vi "Documation.vi"(0 "Max Scale":dbl, 1 "File Nm and format":string, 2 "User/System":string, 3 "Temp":dbl, 4 "Min Scale":dbl) -> (5 "Table":string[][](table))   [LabVIEW 2016]
uses:
  Global Flir-Ax8.vi
  <vilib>/Utility/file.llb/Write Delimited Spreadsheet (string).vi
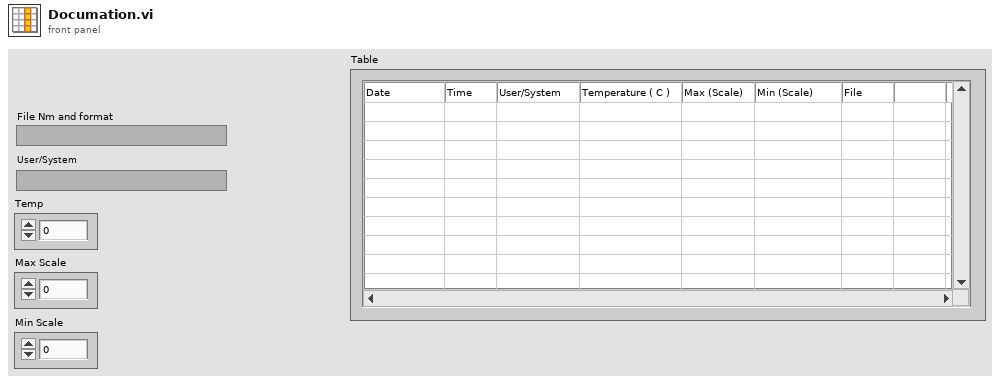
[diagram p1: front panel]
types:
  T1 = enum16{"Check existing file", "create a new file", "write to file", "exit"}
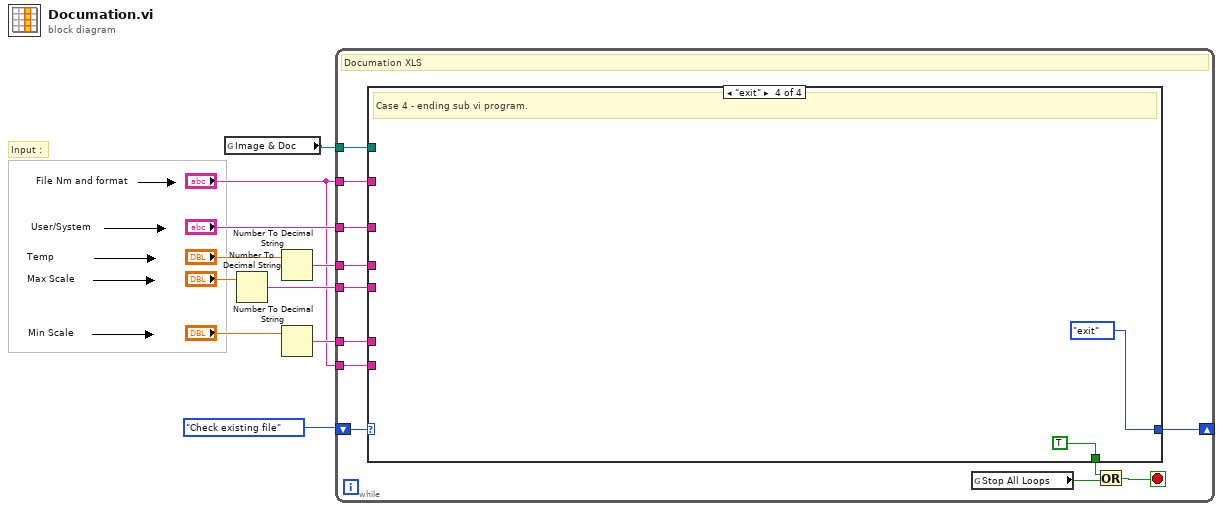
[diagram p0: block diagram]
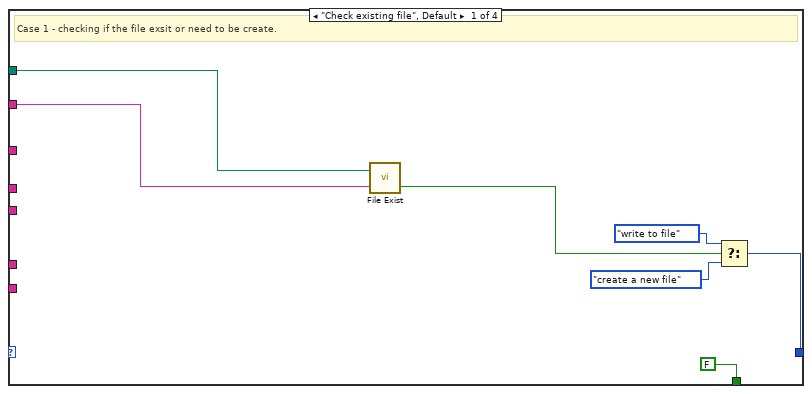
[diagram p2: hidden frame]
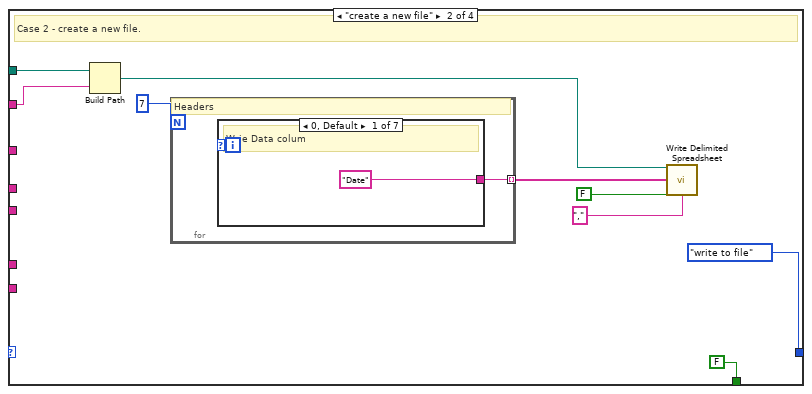
[diagram p3: hidden frame]
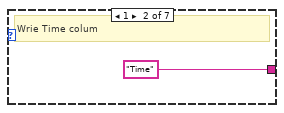
[diagram p4: hidden frame]
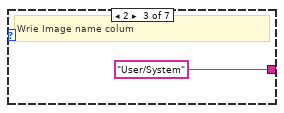
[diagram p5: hidden frame]
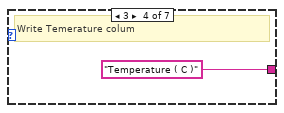
[diagram p6: hidden frame]
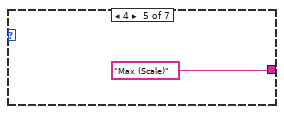
[diagram p7: hidden frame]
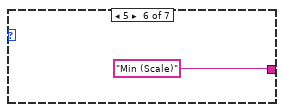
[diagram p8: hidden frame]
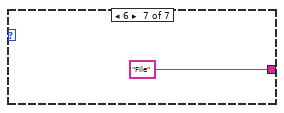
[diagram p9: hidden frame]
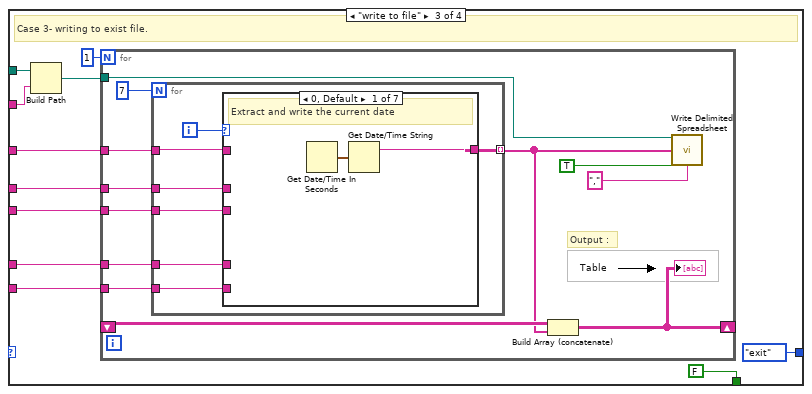
[diagram p10: hidden frame]
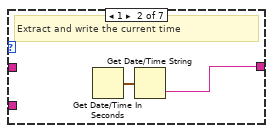
[diagram p11: hidden frame]
diagram:
  # "Input :"
  n1 = global read "Global Flir-Ax8.vi" "Image & Doc"() -> (w1:path)
  n2 = Number To Decimal String(number="Max Scale") -> (decimal integer string=w5:string)  [unwired: 1 in]
  n3 = Number To Decimal String(number="Temp") -> (decimal integer string=w8:string)  [unwired: 1 in]
  n4 = Number To Decimal String(number="Min Scale") -> (decimal integer string=w3:string)  [unwired: 1 in]
  n5 = while {
    shift-right: [w21] -> _
    shift-left: T1."Check existing file" -> [w22]
    tunnel: "User/System" -> [w20]
    tunnel: w1 -> [w19]
    tunnel: "File Nm and format" -> [w18]
    tunnel: w8 -> [w17]
    tunnel: w5 -> [w16]
    tunnel: w3 -> [w15]
    tunnel: "File Nm and format" -> [w14]
    stop <- w11 stop-if-true
    # "Documation XLS"
    n6 = case "Case 1 - checking if the file exsit or need to be create." shown="\"exit\"" w22 {
      tunnel: [w29 T1."write to file" T1."exit" T1."exit"] -> w21
      tunnel: w20 -> [_ _ w57 _]
      tunnel: w19 -> [w28 w34 w56 _]
      tunnel: w18 -> [w24 w33 w55 _]
      tunnel: w17 -> [_ _ w54 _]
      tunnel: w16 -> [_ _ w51 _]
      tunnel: w15 -> [_ _ w50 _]
      tunnel: w14 -> [_ _ w49 _]
      tunnel: [FALSE FALSE FALSE TRUE] -> w12
      frame "Check existing file", Default {
        # "Case 1 - checking if the file exsit or need to be create."
        n7 = call "File Exist.vi"("File Nm"=w24, "File path"=w28) -> ("File Exists"=w25:bool)  [unwired: 1 out]
        n8 = Select(t=T1."write to file", s=w25, f=T1."create a new file") -> (s? t:f=w29:T1)
      }
      frame "create a new file" {
        # "Case 2 - create a new file."
        n9 = Build Path(base path=w34, name or relative path=w33) -> (appended path=w35:path)
        n10 = for {
          N: 7 -> [_]
          tunnel: [w39] -> w38 mode=indexing
          i -> [w40]
          # "Headers"
          n11 = case shown="0, Default" w40 {
            tunnel: ["Date" "Time" "User/System" "Temperature ( C )" "Max (Scale)" "Min (Scale)" "File"] -> w39
            frame 0, Default {
              # "Wrie Data colum"
            }
            frame 1 {
              # "Wrie Time colum"
            }
            frame 2 {
              # "Wrie Image name colum"
            }
            frame 3 {
              # "Write Temerature colum"
            }
            frame 4 {
            }
            frame 5 {
            }
            frame 6 {
            }
          }
        }
        n12 = call-poly <vilib>:"Write Delimited Spreadsheet.vi"("file path (dialog if empty)"=w35, "1D data"=w38, "append to file? (new file:F)"=FALSE, "delimiter (\\t)"="," ("delimiter (\\t)")) -> ()  [unwired: 10 in, 2 out]
      }
      frame "write to file" {
        # "Case 3- writing to exist file."
        n13 = Build Path(base path=w56, name or relative path=w55) -> (appended path=w58:path)
        n14 = for {
          N: 1 -> [_]
          tunnel: w58 -> [w68]
          tunnel: w57 -> [w67]
          tunnel: w54 -> [w66]
          shift-right: [w59] -> _
          shift-left: _ -> [w64]
          tunnel: w51 -> [w62]
          tunnel: w50 -> [w61]
          tunnel: w49 -> [w60]
          # "Output :"
          n15 = for {
            N: 7 -> [_]
            tunnel: [w76] -> w63 mode=indexing
            tunnel: w67 -> [w75]
            tunnel: w66 -> [w74]
            tunnel: w62 -> [w73]
            tunnel: w61 -> [w72]
            tunnel: w60 -> [w71]
            i -> [w77]
            n16 = case shown="0, Default" w77 {
              tunnel: [w78 w80 w82 w83 w84 w85 w86] -> w76
              tunnel: w75 -> [_ _ w82 _ _ _ _]
              tunnel: w74 -> [_ _ _ w83 _ _ _]
              tunnel: w73 -> [_ _ _ _ w84 _ _]
              tunnel: w72 -> [_ _ _ _ _ w85 _]
              tunnel: w71 -> [_ _ _ _ _ _ w86]
              frame 0, Default {
                # "Extract and write the current date"
                n17 = Get Date/Time In Seconds() -> (seconds since 1Jan1904=w79:timestamp)
                n18 = Get Date/Time String(seconds (now)=w79) -> (date string=w78:string)  [unwired: 2 in, 1 out]
              }
              frame 1 {
                # "Extract and write the current time"
                n19 = Get Date/Time In Seconds() -> (seconds since 1Jan1904=w81:timestamp)
                n20 = Get Date/Time String(seconds (now)=w81) -> (time string=w80:string)  [unwired: 2 in, 1 out]
              }
              frame 2 {
                # "insert image name"
              }
              frame 3 {
                # "insert the overstep temerature"
              }
              frame 4 {
                # "insert the max scale temperature"
              }
              frame 5 {
                # "insert the min scale temperature"
              }
              frame 6 {
                # "insert the file name"
              }
            }
          }
          n21 = Build Array (concatenate)(w64, w63) -> (w59:string[][])
          "Table" <- w59
          n22 = call-poly <vilib>:"Write Delimited Spreadsheet.vi"("file path (dialog if empty)"=w68, "1D data"=w63, "append to file? (new file:F)"=TRUE, "delimiter (\\t)"="," ("delimiter (\\t)")) -> ()  [unwired: 10 in, 2 out]
        }
      }
      frame "exit" {
        # "Case 4 - ending sub vi program."
      }
    }
    n23 = global read "Global Flir-Ax8.vi" "Stop All Loops"() -> (w13:bool)
    n24 = Or(x=w12, y=w13) -> (x .or. y?=w11:bool)
  }
